vi "toggle.vi"(11 "Boolean":bool) -> (2 "Boolean 2":bool)   [LabVIEW 2016]
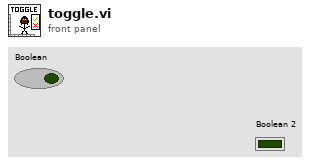
[diagram p1: front panel]
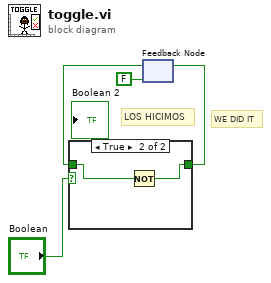
[diagram p0: block diagram]
diagram:
  # "WE DID IT"
  # "LOS HICIMOS"
  n1 = feedback #1(FALSE) -> (w3:bool)
  n2 = case shown="True" "Boolean" {
    tunnel: [w5 w7] -> w2
    tunnel: w3 -> [w5 w6]
    frame False {
    }
    frame True {
      n3 = Not(x=w6) -> (.not. x?=w7:bool)
    }
  }
  n4 = feedback-in #1(w2) -> ()
